vi "readChannelSystemPID.vi"(3 "通道号":i32, 4 "B3":i32, 5 "VISA resource name out 2":refnum<visa-resource-name>) -> (0 "D":dbl, 1 "I":dbl, 2 "P":dbl)   [LabVIEW 2014]
panel:
  out "添加的数组 3":u8[](array[numeric])
  out "添加的数组 2":u8[](array[numeric])
  out "error out":errorcluster
  out "VISA resource name out":refnum<visa-resource-name>
  out "无符号字节数组":u8[](array[numeric])
  out "子字符串":string
  out "p'":dbl
  out "添加的数组":u8[](array[numeric])
  out "返回数":u32
  out "Serial Settings:Number of Bytes at Serial Port":u32
  out "字符串":string
  in  "error out 2":errorcluster caption="error out"
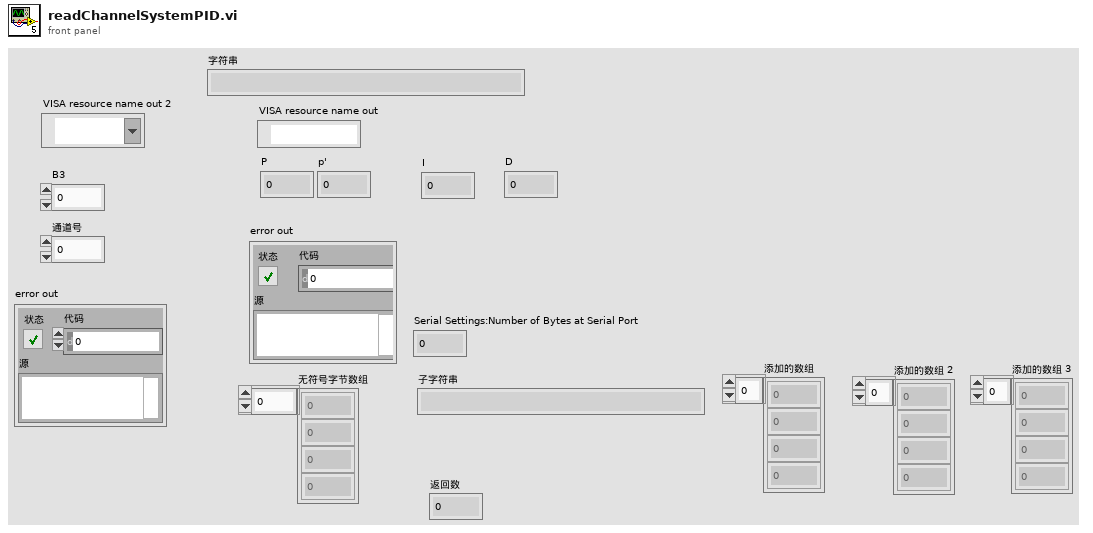
[diagram p1: front panel]
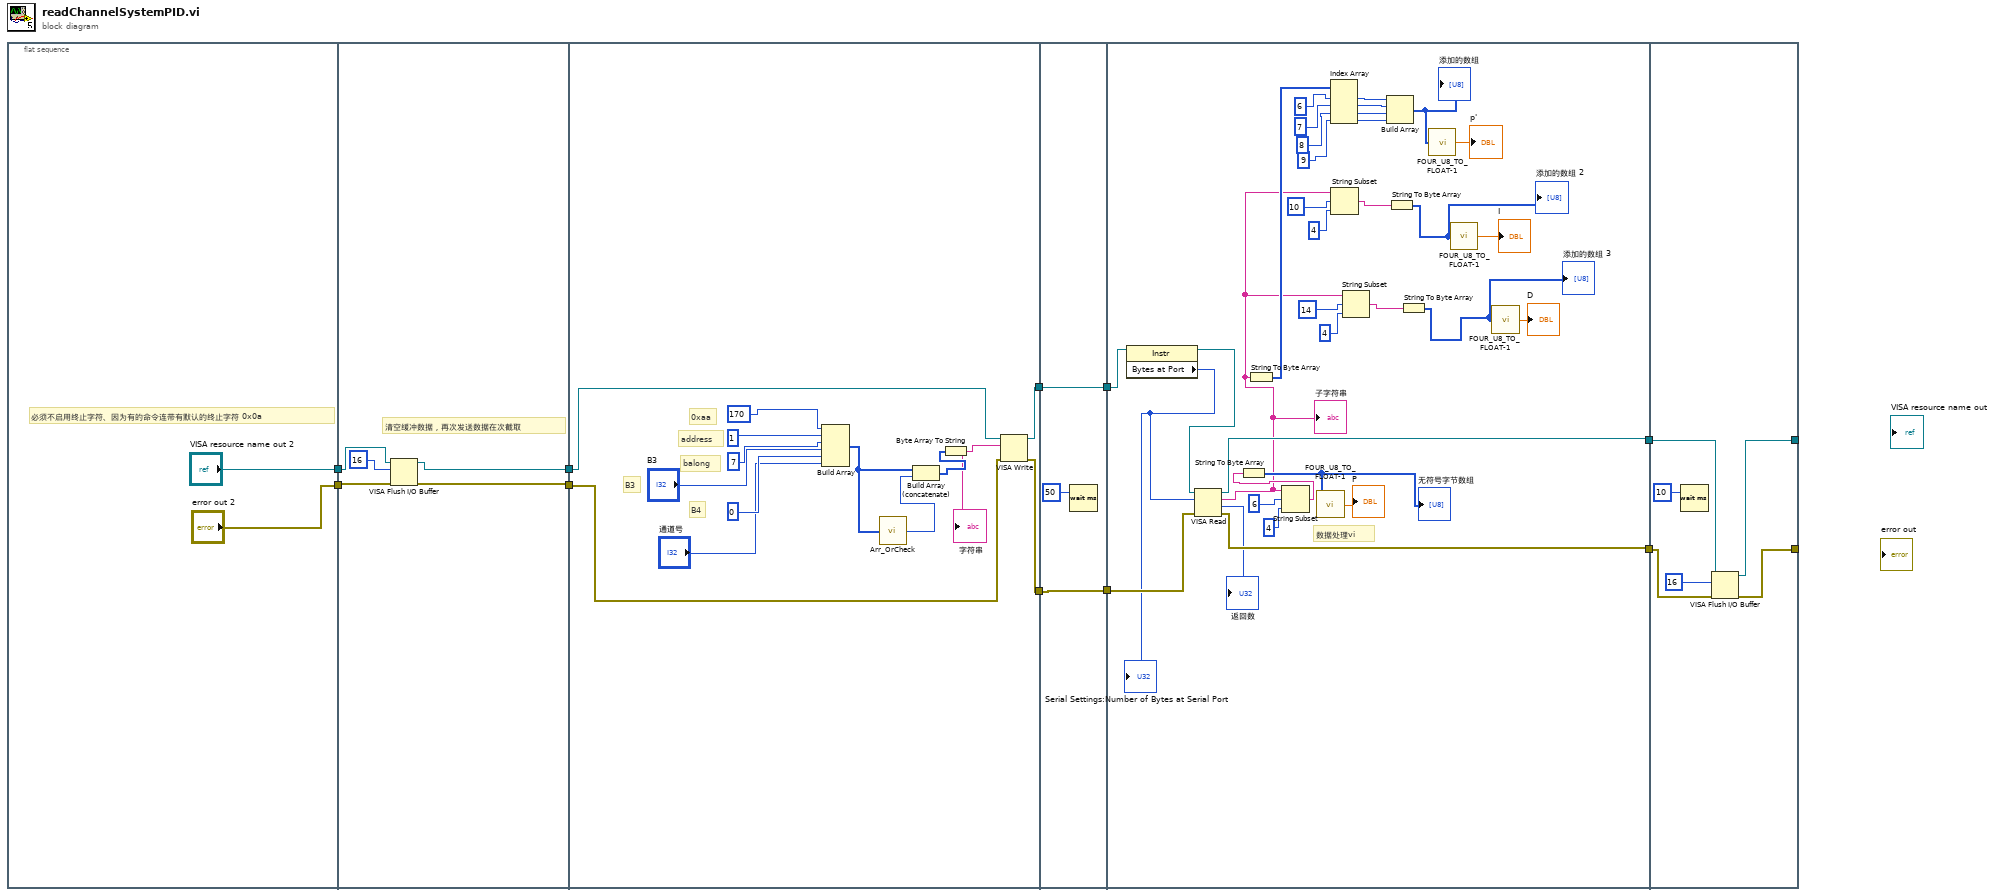
[diagram p0: block diagram]
diagram:
  n1 = flat-sequence {
    tunnel: ["VISA resource name out 2"] -> w10
    tunnel: ["error out 2"] -> w9
    tunnel: w10 -> [w16]
    tunnel: w9 -> [w14]
    tunnel: [w13] -> w8
    tunnel: [w15] -> w7
    tunnel: [w25] -> w6
    tunnel: [w23] -> w5
    tunnel: w8 -> [w24]
    tunnel: w7 -> [w26]
    tunnel: w6 -> [w33]
    tunnel: [w33] -> w4
    tunnel: w5 -> [w32]
    tunnel: [w32] -> w3
    tunnel: w4 -> [w49]
    tunnel: w3 -> [w66]
    tunnel: [w65] -> w2
    tunnel: [w64] -> w1
    tunnel: [w70] -> _
    tunnel: [w69] -> _
    tunnel: w2 -> [w71]
    tunnel: w1 -> [w72]
    frame #0 {
      # "必须不启用终止字符、因为有的命令连带有默认的终止字符 0x0a"
    }
    frame #1 {
      # "清空缓冲数据，再次发送数据在次截取"
      n2 = VISA Flush I/O Buffer(VISA resource name=w16, mask (16)=16, error in (no error)=w14) -> (VISA resource name out=w15:refnum<visa-resource-name>, error out=w13:errorcluster)
    }
    frame #2 {
      # "B4"
      # "B3"
      # "balong"
      # "address"
      # "0xaa"
      n3 = Build Array(170, 1, 7, "B3", 0, "通道号") -> (w22:i32[])
      n4 = call "Arr_OrCheck.vi"("数组"=w22) -> ("抑或的数据值"=w21:u8)
      n5 = Build Array (concatenate)(w22, w21) -> (w20:i32[])
      n6 = Byte Array To String(unsigned byte array=w20) -> (string=w19:string)
      "字符串" <- w19
      n7 = VISA Write(VISA resource name=w26, write buffer=w19, error in (no error)=w24) -> (VISA resource name out=w25:refnum<visa-resource-name>, error out=w23:errorcluster)  [unwired: 1 out]
    }
    frame #3 {
      n8 = Wait (ms)(milliseconds to wait=50) -> ()  [unwired: 1 out]
    }
    frame #4 {
      # "数据处理vi"
      n9 = property class="Instr"(reference=w49) -> (reference out=w48:refnum<visa-resource-name>, "Bytes at Port"=w47:u32)  [unwired: 1 in, 1 out]
      "Serial Settings:Number of Bytes at Serial Port" <- w47
      n10 = VISA Read(VISA resource name=w48, byte count=w47, error in (no error)=w66) -> (VISA resource name out=w64:refnum<visa-resource-name>, read buffer=w35:string, return count=→"返回数":u32, error out=w65:errorcluster)
      "子字符串" <- w35
      n11 = String To Byte Array(string=w35) -> (unsigned byte array=w44:u8[])
      n12 = String Subset(string=w35, offset (0)=6 ("偏移量(0)"), length (rest)=4) -> (substring=w51:string)
      n13 = String To Byte Array(string=w51) -> (unsigned byte array=w68:u8[])
      "无符号字节数组" <- w68
      n14 = call "FOUR_U8_TO_FLOAT-1.vi"("接收数据4*U8"=w68) -> ("输出变量"=→"P":dbl)
      n15 = Index Array(array=w44, index #1=6 ("偏移量(0)"), index #2=7 ("偏移量(0)"), index #3=8 ("偏移量(0)"), index #4=9 ("偏移量(0)")) -> (element #1=w57:u8, element #2=w56:u8, element #3=w55:u8, element #4=w54:u8)
      n16 = String Subset(string=w35, offset (0)=10 ("偏移量(0)"), length (rest)=4) -> (substring=w41:string)
      n17 = String Subset(string=w35, offset (0)=14 ("偏移量(0)"), length (rest)=4) -> (substring=w37:string)
      n18 = Build Array(w57, w56, w55, w54) -> (w53:u8[])
      "添加的数组" <- w53
      n19 = String To Byte Array(string=w41) -> (unsigned byte array=w40:u8[])
      "添加的数组 2" <- w40
      n20 = String To Byte Array(string=w37) -> (unsigned byte array=w36:u8[])
      "添加的数组 3" <- w36
      n21 = call "FOUR_U8_TO_FLOAT-1.vi"("接收数据4*U8"=w53) -> ("输出变量"=→"p'":dbl)
      n22 = call "FOUR_U8_TO_FLOAT-1.vi"("接收数据4*U8"=w40) -> ("输出变量"=→"I":dbl)
      n23 = call "FOUR_U8_TO_FLOAT-1.vi"("接收数据4*U8"=w36) -> ("输出变量"=→"D":dbl)
    }
    frame #5 {
      n24 = Wait (ms)(milliseconds to wait=10) -> ()  [unwired: 1 out]
      n25 = VISA Flush I/O Buffer(VISA resource name=w72, mask (16)=16, error in (no error)=w71) -> (VISA resource name out=w70:refnum<visa-resource-name>, error out=w69:errorcluster)
    }
  }
